vi "AutoThresholdLocalization-3.vi"(5 "[IN] Method":i32(ring) items=["clustering", "entropy", "metric", "moments", "inter-class variance"], 6 "[IN] Autothreshold Images \nInstead Of Generated U8":bool, 7 "[IN] Median Filter":bool, 8 "error IN":errorcluster, 10 "[IN] Binarized Image":T3, 11 "[IN] Source Image":T3) -> (0 "error OUT":errorcluster, 2 "[OUT] X,Y Coordinates":dbl[](array[numeric]))   [LabVIEW 2020]
uses:
  <vilib>/vision/Image Controls.llb/IMAQ Image.ctl
  <vilib>/vision/NI_Vision_Development_Module.lvlib
panel:
  in  "Selection Values":T2(array[cluster])=[{"Measurement Parameter"=22, "Range Lower Value"=10.0, "Range Upper Value"=800.0, "Range"=FALSE, "Measurement Type"=FALSE}] {"Measurement Parameter" items=["Center of Mass X", "Center of Mass Y", "First Pixel X", "First Pixel Y", "Bounding Rect Left", "Bounding Rect Top", "Bounding Rect Right", "Bounding Rect Bottom", "Max Feret Diameter Start X", "Max Feret Diameter Start Y", "Max Feret Diameter End X", "Max Feret Diameter End Y", "Max Horiz. Segment Length Left", "Max Horiz. Segment Length Right", "Max Horiz. Segment Length Row", "-", "Bounding Rect Width", "Bounding Rect Height", "Bounding Rect Diagonal", "Perimeter", "Convex Hull Perimeter", "Holes' Perimeter", "Max Feret Diameter", "Equivalent Ellipse Major Axis", "Equivalent Ellipse Minor Axis", "Equivalent Ellipse Minor Axis (Feret)", "Equivalent Rect Long Side", "Equivalent Rect Short Side", "Equivalent Rect Diagonal", "Equivalent Rect Short Side (Feret)", "Average Horiz. Segment Length", "Average Vert. Segment Length", "Hydraulic Radius", "Waddel Disk Diameter", "-", "Area", "Holes' Area", "Particle & Holes' Area", "Convex Hull Area", "Image Area", "-", "Number of Holes", "Number of Horiz. Segments", "Number of Vert. Segments", "-", "Orientation", "Max Feret Diameter Orientation", "-", "% Area/Image Area", "% Area/(Particle & Holes' Area)", "Ratio of Equivalent Ellipse Axes", "Ratio of Equivalent Rect Sides", "-", "Elongation Factor", "Compactness Factor", "Heywood Circularity Factor", "Type Factor", "-", "Sum X", "Sum Y", "Sum XX", "Sum XY", "Sum YY", "Sum XXX", "Sum XXY", "Sum XYY", "Sum YYY", "-", "Moment of Inertia XX", "Moment of Inertia XY", "Moment of Inertia YY", "Moment of Inertia XXX", "Moment of Inertia XXY", "Moment of Inertia XYY", "Moment of Inertia YYY", "Norm. Moment of Inertia XX", "Norm. Moment of Inertia XY", "Norm. Moment of Inertia YY", "Norm. Moment of Inertia XXX", "Norm. Moment of Inertia XXY", "Norm. Moment of Inertia XYY", "Norm. Moment of Inertia YYY", "Hu Moment 1", "Hu Moment 2", "Hu Moment 3", "Hu Moment 4", "Hu Moment 5", "Hu Moment 6", "Hu Moment 7"]}
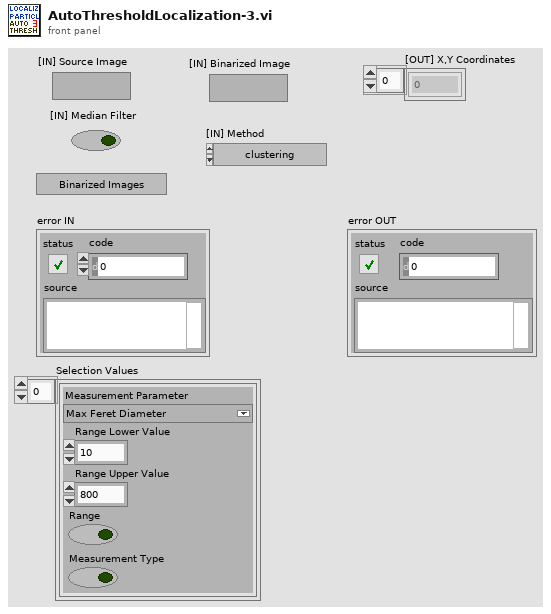
[diagram p1: front panel]
types:
  T1 = typedef "Particle Parameters" = i32
  T2 = cluster{"Measurement Parameter":T1, "Range Lower Value":dbl, "Range Upper Value":dbl, "Range":bool, "Measurement Type":bool}[]
  T3 = typedef "IMAQ Image.ctl" = refnum<image>
  T4 = typedef "Image Type" = u32
  T5 = cluster{"X Size":i32, "Y Size":i32, "Order #":i32}
  T6 = cluster{"Area":dbl, "Number of Holes":dbl, "Bounding Rect":cluster{"Left":dbl, "Top":dbl, "Right":dbl, "Bottom":dbl}, "Center of Mass":cluster{"X":dbl, "Y":dbl}, "Orientation":dbl, "Dimensions":cluster{"Width":dbl, "Height":dbl}}[]
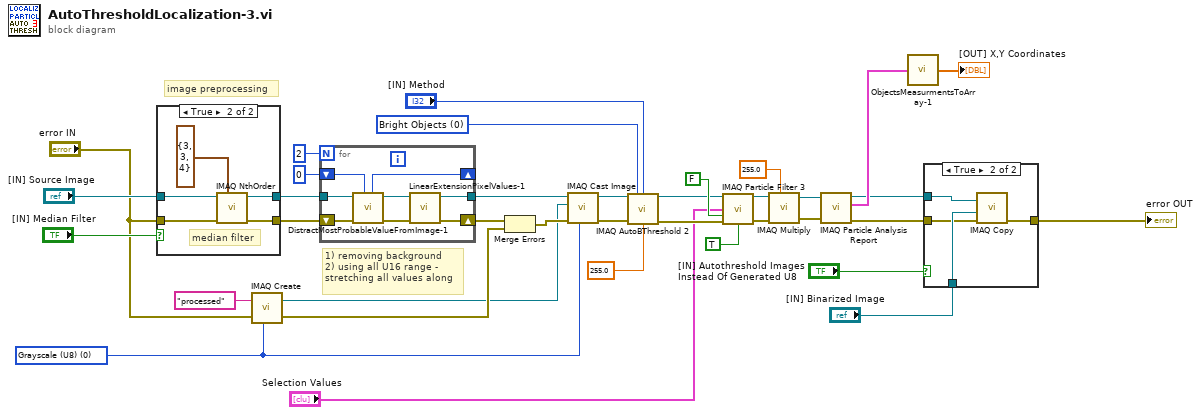
[diagram p0: block diagram]
diagram:
  w23 = u32 0 items=["Bright Objects", "Dark Objects"] ("Look For (Bright Objects)")
  w5 = T4 0 items=["Grayscale (U8)", "Grayscale (I16)", "Grayscale (SGL)", "Complex (CSG)", "RGB (U32)", "HSL (U32)", "RGB (U64)", "Grayscale (U16)"] ("Image Type")
  # "1) removing background\n2) using all U16 range - \nstretching all values along"
  # "image preprocessing"
  n1 = case shown="True" "[IN] Median Filter" {
    tunnel: "[IN] Source Image" -> [w38 w42]
    tunnel: "error IN" -> [w37 w41]
    tunnel: [w38 w40] -> w30
    tunnel: [w37 w39] -> w29
    frame False {
    }
    frame True {
      # "median filter"
      n2 = call "IMAQ NthOrder"("Image Src"=w42, "Size & Order #"=T5 {"X Size"=3, "Y Size"=3, "Order #"=4}, "error in (no error)"=w41) -> ("Image Dst Out"=w40:T3, "error out"=w39:errorcluster)  [unwired: 4 in]
    }
  }
  n3 = call "IMAQ Create"("Image Name"="processed", "Image Type"=w5, "error in (no error)"="error IN") -> ("New Image"=w1:T3, "error out"=w3:errorcluster)  [unwired: 2 in]
  n4 = for {
    N: 2 -> [_]
    shift-right: [w45] -> w4
    shift-left: w29 -> [w49]
    shift-right: [w44] -> _
    shift-left: 0 ("[IN] # Iteration") -> [w51]
    tunnel: w30 -> [w50]
    tunnel: [w46] -> w27
    n5 = call "DistractMostProbableValueFromImage-1.vi"("[IN] # Iteration"=w51, "error in"=w49, "[IN] Max Projected Image"=w50) -> ("error out"=w47:errorcluster, "[OUT] Processed Image"=w48:T3, "[OUT] # Iteration"=w44:i32)  [unwired: 6 in]
    n6 = call "LinearExtensionPixelValues-1.vi"("error in"=w47, "[IN] Max Projected Image"=w48) -> ("error out"=w45:errorcluster, "[OUT] Processed Image"=w46:T3)  [unwired: 8 in]
  }
  n7 = Merge Errors(w4, w3) -> (w2:errorcluster)
  n8 = call "IMAQ Cast Image"("Image Type"=w5, "error in (no error)"=w2, "Image Dst"=w1, "Image Src"=w27) -> ("error out"=w25:errorcluster, "Image Dst Out"=w26:T3)  [unwired: 6 in]
  n9 = call "IMAQ AutoBThreshold 2"("Image Src"=w26, "Look For (Bright Objects)"=w23, "Method (clustering)"="[IN] Method", "error in (no error)"=w25, "Replace Value (1)"=sgl 255.0) -> ("Image Dst Out"=w13:T3, "error out"=w12:errorcluster)  [unwired: 8 in, 1 out]
  n10 = call "IMAQ Particle Filter 3"("Image Src"=w13, "Selection Values"="Selection Values", "Keep/Remove Particles (F)"=FALSE, "error in (no error)"=w12, "Fill Holes? (F)"=TRUE ("Connectivity 4/8 (8)")) -> ("Image Dst Out"=w17:T3, "error out"=w18:errorcluster)  [unwired: 8 in, 1 out]
  n11 = call "IMAQ Multiply"("Image Src A"=w17, "Constant"=255.0, "error in (no error)"=w18) -> ("Image Dst Out"=w16:T3, "error out"=w15:errorcluster)  [unwired: 4 in]
  n12 = call "IMAQ Particle Analysis Report"("error in (no error)"=w15, "Image"=w16) -> ("error out"=w10:errorcluster, "Particle Reports (Pixels)"=w11:T6, "Image Out (duplicate)"=w9:T3)  [unwired: 4 in, 3 out]
  n13 = call "ObjectsMeasurmentsToArray-1.vi"("[IN] Particle Reports (Pixels)"=w11) -> ("[OUT] X,Y Coordinates"=→"[OUT] X,Y Coordinates":dbl[])
  n14 = case shown="True" "[IN] Autothreshold Images \nInstead Of Generated U8" {
    tunnel: w10 -> [w52 w54]
    tunnel: [w52 w56] -> w32
    tunnel: w9 -> [_ w53]
    tunnel: "[IN] Binarized Image" -> [_ w55]
    frame False {
    }
    frame True {
      n15 = call "IMAQ Copy"("error in (no error)"=w54, "Image Dst"=w55, "Image Src"=w53) -> ("error out"=w56:errorcluster)  [unwired: 3 in, 1 out]
    }
  }
  "error OUT" <- w32
